vi "ExtractElement.vi"(10 "subimage in":refnum<vi>, 11 "acquisition frame":T1) -> (1 "extracted image":u8[][](array[numeric]), 3 "full image":u8[][](array[numeric]))   [LabVIEW 2018]
uses:
  typedef/AcquisitionFrame.ctl
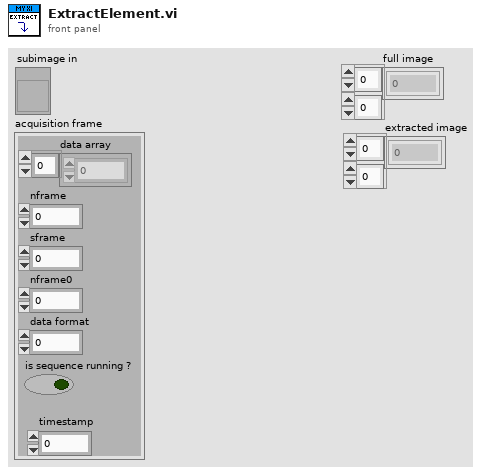
[diagram p1: front panel]
types:
  T1 = typedef "AcquisitionFrame.ctl" = cluster{"data array":u8[], "nframe":i32, "sframe":i32, "nframe0":i32, "data format":i32, "is sequence running ?":bool, "timestamp":dbl}
  T2 = typedef "LVPointDoubleTypeDef.ctl" = cluster{"X":dbl, "Y":dbl}
  T3 = cluster{"2^n : x":i8, "2^n : y":i8, "lower left box Position":T2, "Height":i32, "Width":i32}
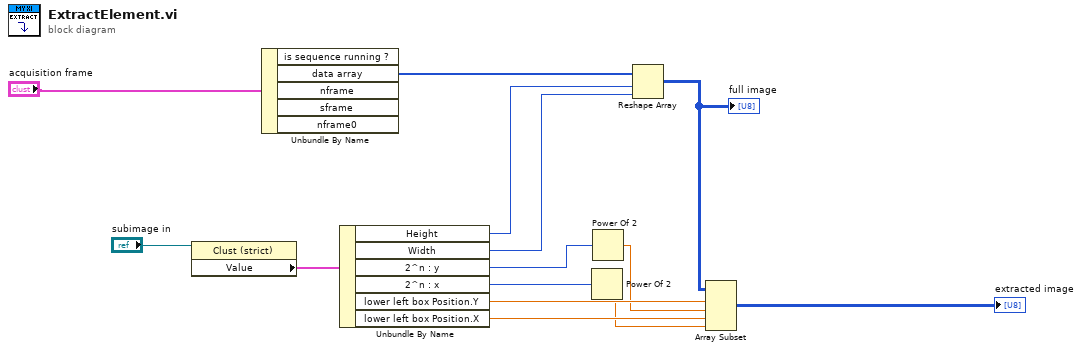
[diagram p0: block diagram]
diagram:
  n1 = property on="Property Node" class="Clust (strict)"(reference="subimage in") -> ("Value"=w12:T3)  [unwired: 1 in, 2 out]
  n2 = Unbundle By Name("acquisition frame") -> ("data array"=w14:u8[])  [unwired: 4 out]
  n3 = Unbundle By Name(w12) -> ("Height"=w4:i32, "Width"=w3:i32, "2^n : y"=w11:i8, "2^n : x"=w10:i8, "lower left box Position.Y"=w9:dbl, "lower left box Position.X"=w8:dbl)
  n4 = Power Of 2(x=w10) -> (2^x=w6:dbl)
  n5 = Power Of 2(x=w11) -> (2^x=w7:dbl)
  n6 = Reshape Array "Reshape Array"(w14, w4, w3) -> (w5:u8[][])
  "full image" <- w5
  n7 = Array Subset(array=w5, index (row)=w9, length (row)=w7, index (col)=w8, length (col)=w6) -> (→"extracted image":u8[][])
